vi "SendDataToServer.vi"(8 "error in (no error)":errorcluster, 9 "data":variant, 10 "Query_type":T1, 11 "Gviewer in":refnum<class "Gviewer.lvclass">) -> (0 "error out":errorcluster, 3 "Gviewer out":refnum<class "Gviewer.lvclass">)   [LabVIEW 2020, in "Sgraph_lib_V1.lvlib" / "Gviewer.lvclass"]
doc: "Andre Koelewijn, 5 jan 2021\n\nSend Request to Gserver Queue"
uses:
  Gviewer.lvclass
  Gserver/controls/Typedef_QueryType.ctl
  Gserver/controls/Typedef_Gviewer-Query.ctl
  Gviewer.lvclass/Gviewer.ctl
  Gserver/Gserver.lvclass
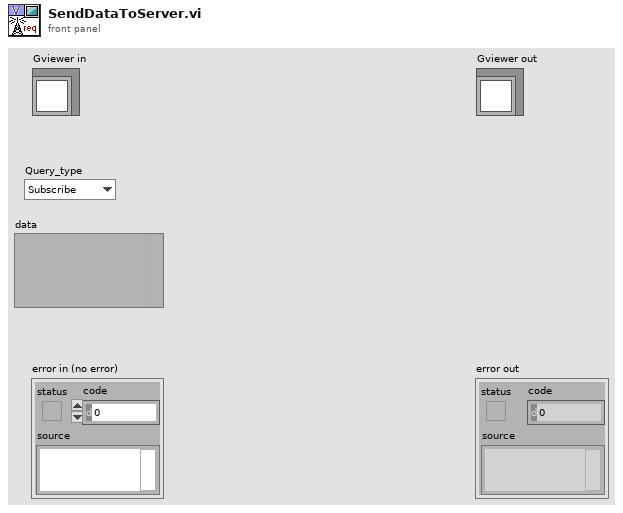
[diagram p1: front panel]
types:
  T1 = typedef "Sgraph_lib_V1.lvlib/Gserver.lvclass/Typedef_QueryType.ctl" = enum16{"Subscribe", "DataRequest", "RequestAllTags", "RequestIniPath", "FAMMstarted", "SetClientOptions", "GviewerUpdate", "OpenNewGraph", "CloseClient", "CloseAllClients", "Close Gserver", "OpenMemoryMap", "MeMapDataRequest", "MeMapDataResponse", "OpenDBeditor", "CheckDBeditorRunning", "StoppedDBeditor", "SaveDB_TAGpropRecord", "ConfirmDB_TAGpropSave"}
  T2 = typedef "Sgraph_lib_V1.lvlib/Gserver.lvclass/Typedef_Gviewer-Query.ctl" = cluster{"Query_type":T1, "data":variant, "Source":string, "Time Stamp":timestamp}
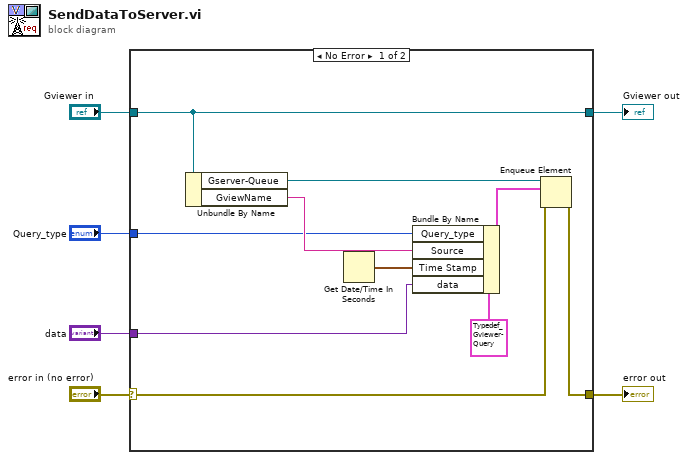
[diagram p0: block diagram]
diagram:
  n1 = case shown="No Error" "error in (no error)" {
    selector: "error in (no error)" -> [w10 w18]
    tunnel: [w9 w18] -> w5
    tunnel: [w11 w17] -> w3
    tunnel: "Gviewer in" -> [w11 w17]
    tunnel: "Query_type" -> [w8 _]
    tunnel: "data" -> [w7 _]
    frame No Error {
      n2 = Unbundle By Name(w11) -> ("Gserver-Queue"=w16:refnum<queue>, "GviewName"=w14:string)
      n3 = Get Date/Time In Seconds() -> (seconds since 1Jan1904=w13:timestamp)
      n4 = Bundle By Name(cluster=T2 {"Query_type"=enum."Subscribe", "data"=variant, "Source"="", "Time Stamp"=timestamp(0 s since 1904-01-01)} ("element"), "Query_type"=w8, "Source"=w14, "Time Stamp"=w13, "data"=w7) -> (w15:T2)
      n5 = Enqueue Element(queue=w16, element=w15, error in (no error)=w10) -> (error out=w9:errorcluster)  [unwired: 1 in, 2 out]
    }
    frame Error {
    }
  }
  "error out" <- w5
  "Gviewer out" <- w3
